vi "CreateDefectFile.vi"(4 "Region":u16, 6 "Segment:":string, 7 "Pass rate":dbl format="%.2f", 8 "Defect description list":i32[](array[numeric]), 9 "Bad channel array":i32[](array[numeric]), 10 "No of bad strips":i32, 11 "Filename IN":string) -> (0 "DBfileSaved?":bool, 1 "passed":bool, 3 "DBFileName OUT":string)   [LabVIEW 2018]
uses:
  general_VIs/globals/QC_RunInformation.vi
  general_VIs/globals/QC_MeasurementSetup.vi
panel:
  in  "Pathname IN":string
  in  "inspect":bool
  in  "stop":bool
  in  "?":bool
  in  "cancel":bool
  in  "create file":bool
  out "% good strips:":dbl format="%.2f"
  out "Date:":string
  out "Location:":string
  out "Operator:":string
  out "Passed?":bool
  out "ITk Serial No.:":string
  out "Comments?":string
  in  "Problem?":bool
  in  "Bad channel list":i32(listbox)
  # "Write Strip Defect DataBase File"
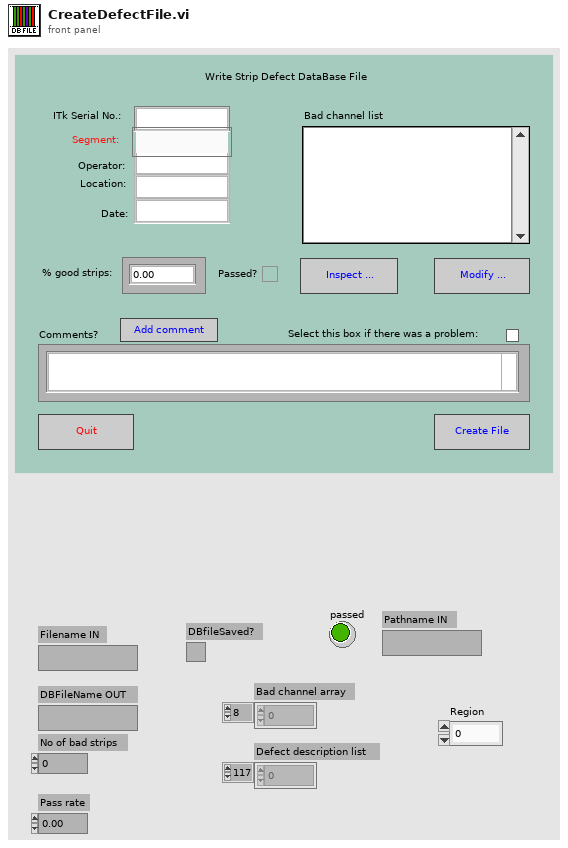
[diagram p1: front panel]
types:
  T1 = cluster{"Institute":string, "Manufacturers":string[], "Devices":string[], "Serialnumbers Lookup DB":string, "Data directory":string, "Backup & screenshot directory":string, "List of known users":string[]}
  T2 = cluster{"Sensor Serial No.:":string, "Wafer Serial No.:":string, "Batch:":string, "Manufacturer:":string, "Device Category:":string, "Database Serial No.:":string, "Initiated:":string, "Test":string, "Instruments used:":string, "Probeplan used:":string, "End of Run comment:":string, "User:":string}
  T3 = enum16{"open", "open or create", "create or replace", "create"}
  T4 = cluster{"Bias Supply":refnum<class "SupplyControl.lvclass">, "SMU":refnum<class "SupplyControl.lvclass">, "LCR":refnum<class "LCRControl.lvclass">, "Probe Card Channels":i32, "Bias Voltage [V]":dbl, "First strip":i32, "Last strip":i32, "Base Voltage [V]":dbl, "Base Ramp Step [V]":dbl, "Base Ramp Interval [ms]":u32, "High Voltage [V]":dbl, "High Ramp Step [V]":dbl, "High Ramp Interval [ms]":u32, "Single Needle":bool, "Temperature Readout":enum16{"Read Arduino", "Enter manually"}, "Arduino":refnum<class "ArduinoControl.lvclass">, "Fraction of good strips [%]":dbl, "ProbeStation":refnum<class "ProbeStationControl.lvclass">, "AC frequency [Hz]":i32, "Switching":refnum<class "Switching.lvclass">, "Matrix used?":bool, "Matrix X Channels":cluster{"Bias Supply / SMU LO":i32, "Bias Supply / SMU HI":i32, "CV Box LO":i32, "CV Box HI":i32, "CV Box LO IN":i32, "CV Box HI IN":i32, "Volt meter LO":i32, "Volt meter HI":i32, "Mux1 C1":i32, "Mux1 C2":i32, "Mux2 C1":i32, "Mux2 C2":i32}, "Pinholes Y/N":bool, "Capacitance Y/N":bool, "Resistance Y/N":bool}
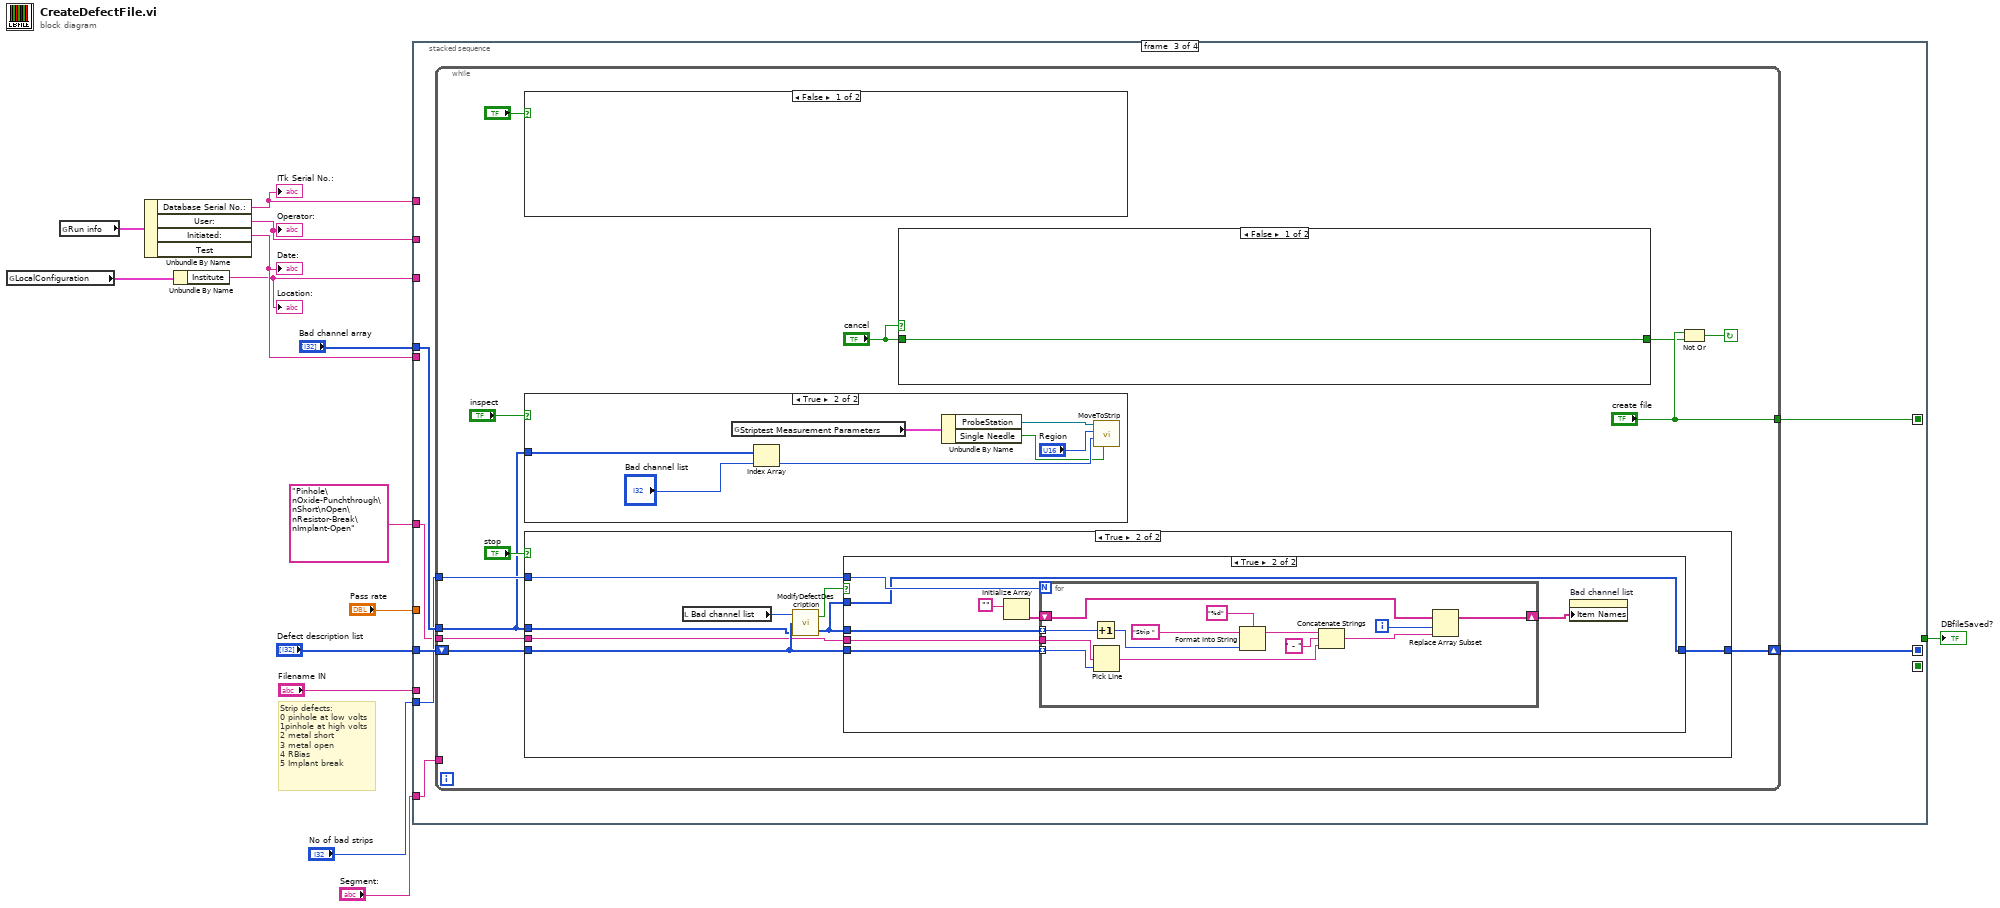
[diagram p0: block diagram]
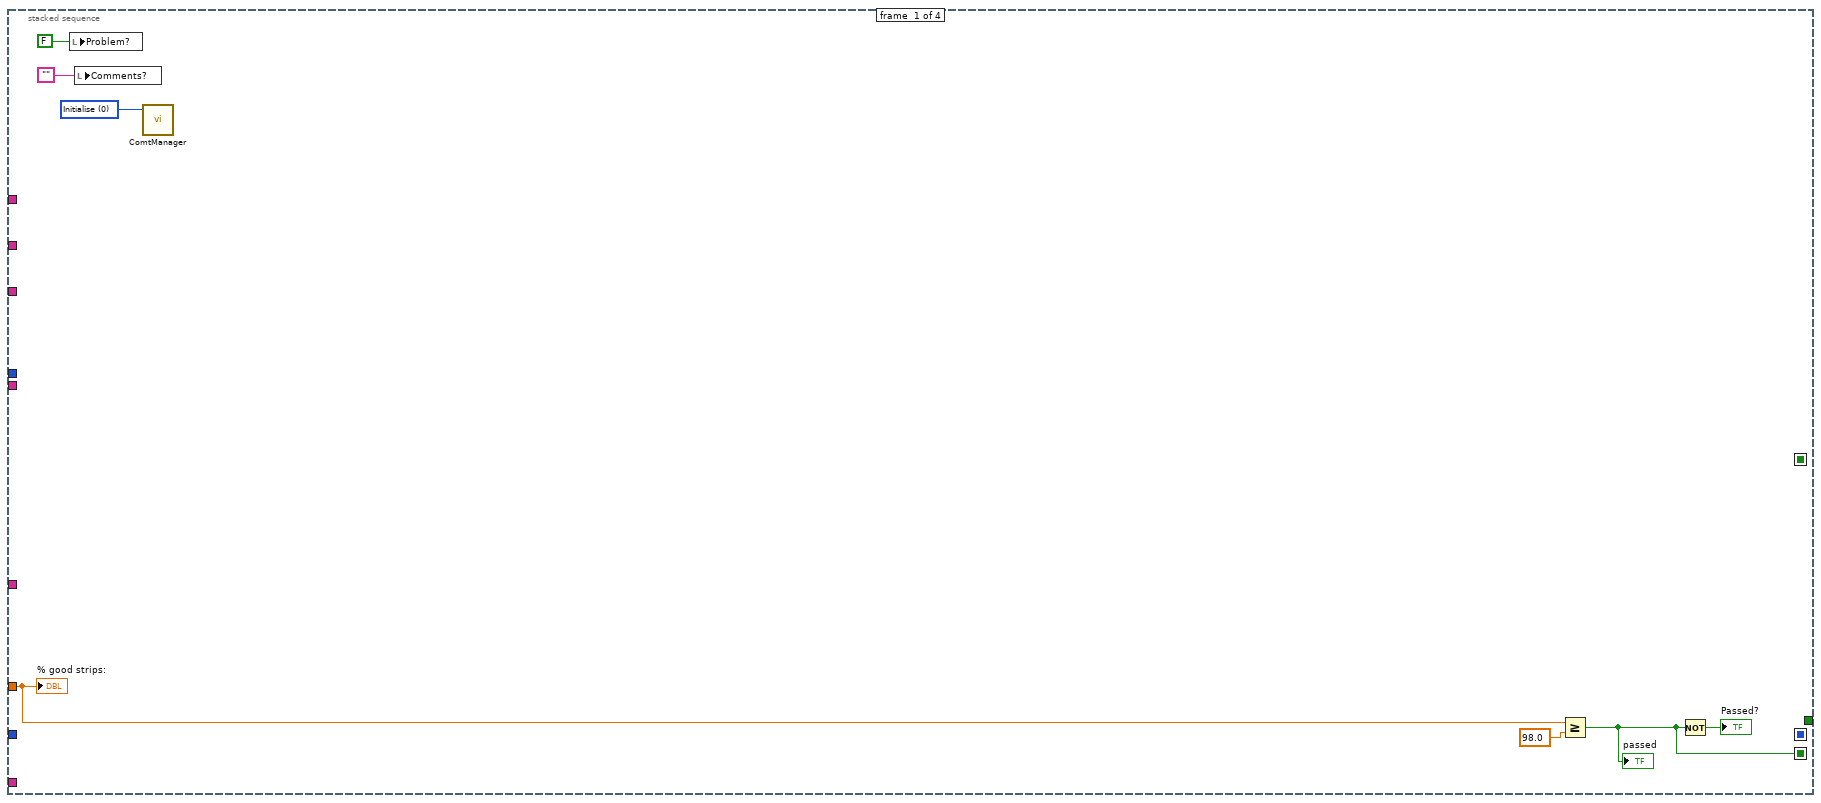
[diagram p2: hidden frame]
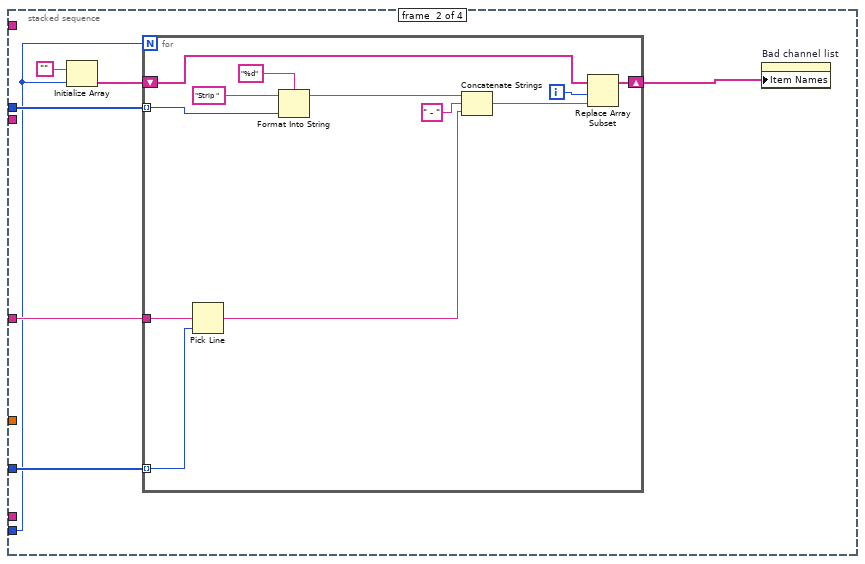
[diagram p3: hidden frame]
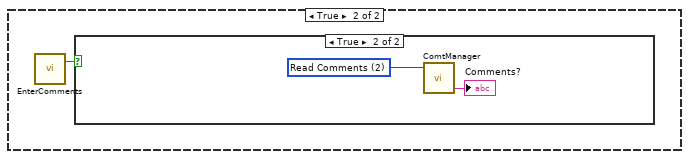
[diagram p7: hidden frame]
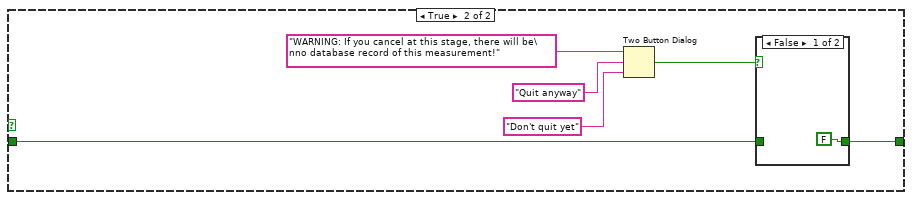
[diagram p9: hidden frame]
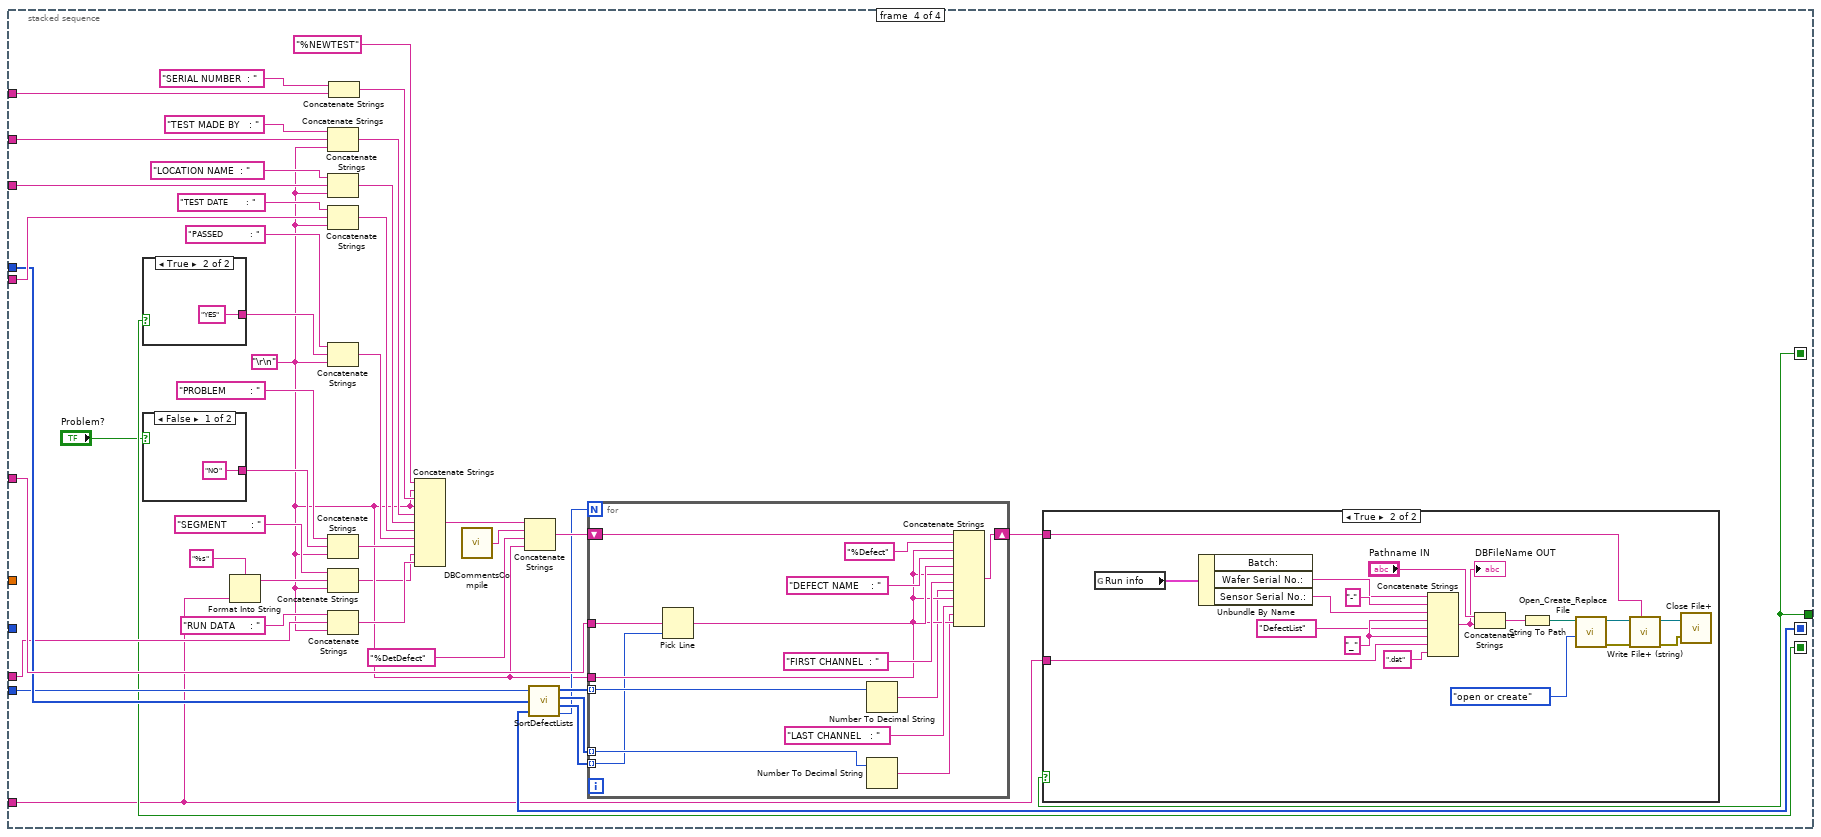
[diagram p11: hidden frame]
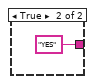
[diagram p13: hidden frame]
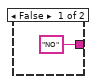
[diagram p14: hidden frame]
diagram:
  # "Strip defects:\n0 pinhole at low volts\n1pinhole at high volts\n2 metal short\n3 metal open\n4 RBias\n5 Implant break"
  n1 = global read "QC_RunInformation.vi" "LocalConfiguration"() -> (w2:T1)
  n2 = global read "QC_RunInformation.vi" "Run info"() -> (w13:T2)
  n3 = Unbundle By Name(w13) -> ("Database Serial No.:"=w12:string, "User:"=w11:string, "Initiated:"=w10:string)  [unwired: 1 out]
  "ITk Serial No.:" <- w12
  "Operator:" <- w11
  "Date:" <- w10
  n4 = Unbundle By Name(w2) -> ("Institute"=w1:string)
  "Location:" <- w1
  n5 = stacked-sequence {
    seq-local: [w15 _ _ _] -> [_ _ _ w117]
    seq-local: [_ _ w47 _] -> [_ _ _ w135]
    seq-local: [_ _ w44 _] -> [_ _ _ w125]
    tunnel: "No of bad strips" -> [_ w22 w43 w119]
    tunnel: "Bad channel array" -> [_ w25 w46 w124]
    tunnel: "Pinhole\nOxide-Punchthrough\nShort\nOpen\nResistor-Break\nImplant-Open" -> [_ w26 w41 w137]
    tunnel: w12 -> [_ _ _ w130]
    tunnel: w11 -> [_ _ _ w142]
    tunnel: w10 -> [_ _ _ w141]
    tunnel: w1 -> [_ _ _ w140]
    tunnel: [_ _ _ w135] -> w9
    tunnel: "Filename IN" -> [_ _ _ w118]
    tunnel: "Defect description list" -> [_ w24 w45 _]
    tunnel: "Pass rate" -> [w17 _ _ _]
    tunnel: "Segment:" -> [_ _ w42 w110]
    frame #0 {
      w16 = u16 0 items=["Initialise", "Add comment", "Read Comments"] ("Action")
      n6 = local write "Problem?"(FALSE ("Problem?")) -> ()
      n7 = local write "Comments?"("") -> ()
      n8 = call "ComtManager.vi"("Action"=w16) -> ()  [unwired: 2 in, 3 out]
      n9 = Greater Or Equal?(x=w17, y=98.0) -> (x >= y?=w15:bool)
      "passed" <- w15
      n10 = Not(x=w15) -> (.not. x?=→"Passed?":bool)
      "% good strips:" <- w17
    }
    frame #1 {
      n11 = Initialize Array("", w22) -> (w27:string[])
      n12 = for {
        N: w22 -> [_]
        shift-right: [w35] -> w23
        shift-left: w27 -> [w38]
        tunnel: w25 -> [w29] mode=indexing
        tunnel: w26 -> [w34]
        tunnel: w24 -> [w30] mode=indexing
        i -> [w37]
        n13 = Pick Line(multi-line string=w34, line index=w30) -> (output string=w31:string)  [unwired: 1 in]
        n14 = Format Into String(format string="%d", initial string="Strip ", w29) -> (resulting string=w33:string)  [unwired: 1 in, 1 out]
        n15 = Concatenate Strings(w33, " - ", w31) -> (w36:string)
        n16 = Replace Array Subset(array=w38, new element=w36, index=w37) -> (w35:string[])
      }
      n17 = property on="Bad channel list" class="LstBox (strict)"("Item Names"=w23) -> ()  [unwired: 2 in, 2 out]
    }
    frame #2 {
      n18 = while {
        tunnel: ["create file"] -> w47
        tunnel: w46 -> [w49]
        shift-right: [w52] -> w44
        shift-left: w45 -> [w53]
        tunnel: w43 -> [w51]
        tunnel: w42 -> [_]
        tunnel: w41 -> [w48]
        stop <- w59 continue-if-true
        n19 = case shown="False" "?" {
          frame False {
          }
          frame True {
            n20 = call "EnterComments.vi"() -> ("update?"=w98:bool)  [unwired: 4 in]
            n21 = case shown="True" w98 {
              frame False {
              }
              frame True {
                w100 = u16 2 items=["Initialise", "Add comment", "Read Comments"] ("Action")
                n22 = call "ComtManager.vi"("Action"=w100) -> ("Comment out"=→"Comments?":string)  [unwired: 2 in, 2 out]
              }
            }
          }
        }
        n23 = case shown="True" "inspect" {
          tunnel: w49 -> [_ w66]
          frame False {
          }
          frame True {
            n24 = global read "QC_MeasurementSetup.vi" "Striptest Measurement Parameters"() -> (w62:T4)
            n25 = Index Array(array=w66, index="Bad channel list") -> (element=w64:i32)
            n26 = Unbundle By Name(w62) -> ("ProbeStation"=w61:refnum<class "ProbeStationControl.lvclass">, "Single Needle"=w63:bool)
            n27 = call "MoveToStrip.vi"("Single Needle"=w63, "Strip No."=w64, "Region"="Region", "ProbeStationControl in"=w61) -> ()  [unwired: 5 in, 3 out]
          }
        }
        n28 = case shown="True" "stop" {
          tunnel: w53 -> [w67 w73]
          tunnel: w49 -> [_ w71]
          tunnel: [w67 w72] -> w52
          tunnel: w51 -> [_ w70]
          tunnel: w48 -> [_ w69]
          frame False {
          }
          frame True {
            n29 = local read "Bad channel list"() -> (w75:i32)
            n30 = call "ModifyDefectDescription.vi"("Bad Channel array"=w71, "Defect flag array"=w73, "Defect Number"=w75) -> ("Defect flag array out"=w68:i32[], "Updated?"=w74:bool)
            n31 = case shown="True" w74 {
              tunnel: w73 -> [w76 w79]
              tunnel: [w76 w77] -> w72
              tunnel: w68 -> [_ w78]
              tunnel: w70 -> [_ w80]
              tunnel: w69 -> [_ w81]
              tunnel: w68 -> [_ w77]
              frame False {
              }
              frame True {
                n32 = Initialize Array("") -> (w83:string[])  [unwired: 1 in]
                n33 = for {
                  N: w80 -> [_]
                  shift-right: [w92] -> w82
                  shift-left: w83 -> [w95]
                  tunnel: w78 -> [w85] mode=indexing
                  tunnel: w81 -> [w91]
                  tunnel: w79 -> [w87] mode=indexing
                  i -> [w94]
                  n34 = Increment(x=w85) -> (x+1=w86:i32)
                  n35 = Pick Line(multi-line string=w91, line index=w87) -> (output string=w88:string)  [unwired: 1 in]
                  n36 = Format Into String(format string="%d", initial string="Strip ", w86) -> (resulting string=w90:string)  [unwired: 1 in, 1 out]
                  n37 = Concatenate Strings(w90, " - ", w88) -> (w93:string)
                  n38 = Replace Array Subset(array=w95, new element=w93, index=w94) -> (w92:string[])
                }
                n39 = property on="Bad channel list" class="LstBox (strict)"("Item Names"=w82) -> ()  [unwired: 2 in, 2 out]
              }
            }
          }
        }
        n40 = case shown="False" "cancel" {
          tunnel: [w101 w103] -> w57
          tunnel: "cancel" -> [w101 w102]
          frame False {
          }
          frame True {
            n41 = Two Button Dialog(message="WARNING: If you cancel at this stage, there will be\nno database record of this measurement!", 1:"Don't quit yet" ("F button name (\"Cancel\")"), 2:"Quit anyway" ("T button name (\"OK\")")) -> (T button?=w104:bool)
            n42 = case shown="False" w104 {
              tunnel: [FALSE w109] -> w103
              tunnel: w102 -> [_ w109]
              frame False {
              }
              frame True {
              }
            }
          }
        }
        n43 = Not Or(1:w57, 2:"create file") -> (0:w59:bool)
      }
    }
    frame #3 {
      w112 = "\r\n"
      n44 = case shown="True" w117 {
        tunnel: ["NO" "YES"] -> w139
        frame False {
        }
        frame True {
        }
      }
      n45 = case shown="False" "Problem?" {
        tunnel: ["NO" "YES"] -> w138
        frame False {
        }
        frame True {
        }
      }
      n46 = Format Into String(format string="%s", w110) -> (resulting string=w113:string)  [unwired: 2 in, 1 out]
      n47 = Concatenate Strings("TEST MADE BY   : ", w142, w112) -> (w147:string)
      n48 = Concatenate Strings("LOCATION NAME  : ", w140, w112) -> (w146:string)
      n49 = Concatenate Strings("TEST DATE      : ", w141, w112) -> (w145:string)
      n50 = Concatenate Strings("PASSED         : ", w139, w112) -> (w144:string)
      n51 = Concatenate Strings("PROBLEM        : ", w138, w112) -> (w143:string)
      n52 = Concatenate Strings("SEGMENT        : " ("string"), w113, w112) -> (w111:string)
      n53 = Concatenate Strings("RUN DATA     : ", w118, w112) -> (w133:string)
      n54 = Concatenate Strings("SERIAL NUMBER  : ", w130) -> (w132:string)
      n55 = Concatenate Strings("%NEWTEST", w112, w132, w112, w147, w146, w145, w144, w143, w111, w133) -> (w127:string)
      n56 = call "DBCommentsCompile.vi"() -> ("Comments out"=w126:string)
      n57 = Concatenate Strings(w127, w126, "%DetDefect", w112) -> (w129:string)
      n58 = call "SortDefectLists.vi"("No of bad strips"=w119, "Defect strips IN"=w124, "Defect flag array IN"=w125) -> ("First defect No"=w122:i32[], "Last Defect No"=w121:i32[], "Defect Flag array OUT"=w123:i32[], "No of database entries"=w120:i32)
      n59 = for {
        N: w120 -> [_]
        shift-right: [w178] -> w136
        shift-left: w129 -> [w179]
        tunnel: w112 -> [w177]
        tunnel: w137 -> [w183]
        tunnel: w123 -> [w174] mode=indexing
        tunnel: w122 -> [w176] mode=indexing
        tunnel: w121 -> [w175] mode=indexing
        n60 = Pick Line(multi-line string=w183, line index=w174) -> (output string=w182:string)  [unwired: 1 in]
        n61 = Number To Decimal String(number=w176) -> (decimal integer string=w173:string)  [unwired: 1 in]
        n62 = Number To Decimal String(number=w175) -> (decimal integer string=w172:string)  [unwired: 1 in]
        n63 = Concatenate Strings(w179, "%Defect", w177, "DEFECT NAME    : ", w182, w177, "FIRST CHANNEL  : ", w173, w177, "LAST CHANNEL   : ", w172, w177) -> (w178:string)
      }
      n64 = case shown="True" w135 {
        tunnel: w136 -> [_ w166]
        tunnel: w110 -> [_ w155]
        frame False {
        }
        frame True {
          w157 = "_"
          n65 = global read "QC_RunInformation.vi" "Run info"() -> (w165:T2)
          n66 = Unbundle By Name(w165) -> ("Wafer Serial No.:"=w163:string, "Sensor Serial No.:"=w162:string)  [unwired: 1 out]
          n67 = Concatenate Strings(w163, "-", w162, w157, "DefectList", w157, w155, ".dat") -> (w160:string)
          "DBFileName OUT" <- w160
          n68 = Concatenate Strings("Pathname IN", w160) -> (w159:string)
          n69 = String To Path(string=w159) -> (path=w158:path)
          n70 = call <vilib>:"Open_Create_Replace File.vi"("function (open:0)"=T3."open or create", "file path"=w158) -> ("error out"=w168:errorcluster, "refnum"=w170:refnum<file>)  [unwired: 6 in, 2 out]
          n71 = call <vilib>:"Write File+ (string).vi"("string"=w166, "error in (no error)"=w168, "refnum"=w170) -> ("error out"=w167:errorcluster, "dup refnum"=w169:refnum<file>)  [unwired: 4 in, 1 out]
          n72 = call <vilib>:"Close File+.vi"("error in (no error)"=w167, "refnum"=w169) -> ()  [unwired: 3 in, 3 out]
        }
      }
    }
  }
  "DBfileSaved?" <- w9
